vi "Producto.vi"(8 "error in (no error)":errorcluster, 9 "valor actual":u16, 10 "Item Names":string[][](array[string]), 11 "Coffee Actor in":refnum<class "Coffee Actor.lvclass">) -> (0 "error out":errorcluster, 3 "Coffee Actor out":refnum<class "Coffee Actor.lvclass">)   [LabVIEW 2019, in "Coffee Actor.lvlib" / "Coffee Actor.lvclass"]
uses:
  Coffee Actor.lvclass
  Coffee Actor.lvclass/Coffee Actor.ctl
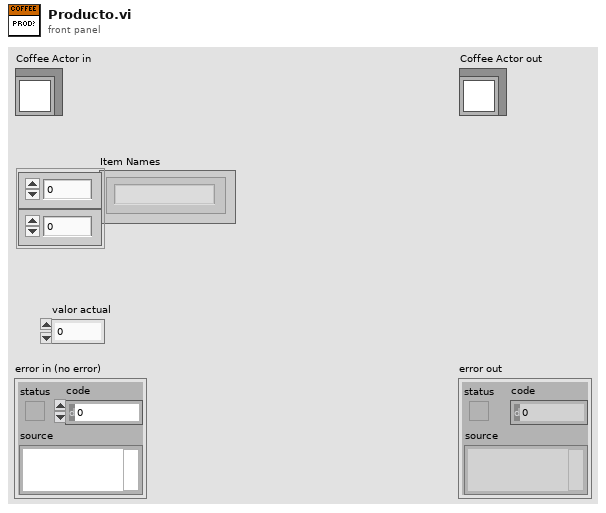
[diagram p1: front panel]
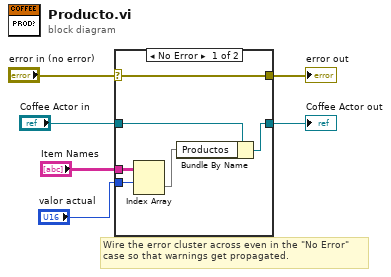
[diagram p0: block diagram]
diagram:
  # "Wire the error cluster across even in the \"No Error\"\ncase so that warnings get propagated."
  n1 = case shown="No Error" "error in (no error)" {
    selector: "error in (no error)" -> [w12 w14]
    tunnel: [w12 w14] -> w5
    tunnel: [w10 w13] -> w3
    tunnel: "Coffee Actor in" -> [w11 w13]
    tunnel: "Item Names" -> [w9 _]
    tunnel: "valor actual" -> [w8 _]
    frame No Error {
      n2 = Index Array(array=w9, index (row)=w8) -> (element=w7:string[])  [unwired: 1 in]
      n3 = Bundle By Name(cluster=w11, "Productos"=w7) -> (w10:refnum<class "Coffee Actor.lvclass">)
    }
    frame Error {
    }
  }
  "error out" <- w5
  "Coffee Actor out" <- w3
